vi "Measure-combined.vi"(7 "LaserResponse in":refnum<class "MC-LaserResponse.lvclass">, 8 "error in (no error)":errorcluster, 9 "Device index":i32, 10 "File path":path, 11 "SM1000-control in":T1) -> (0 "error out":errorcluster, 3 "SM1000-control out":T1, 5 "LaserResponse":refnum<class "MC-LaserResponse.lvclass">)   [LabVIEW 2013, in "MaterialCharacterization.lvlib" / "MC-SM1000.lvclass"]
uses:
  MC-SM1000.lvclass
  Object-reference.ctl
  LaserPulseAnalyser/MC-LaserResponse.lvclass
  <vilib>/DAQmx/read.llb/DAQmx Read (Digital 1D U32 1Chan NSamp).vi
  <vilib>/DAQmx/read.llb/DAQmx Read (Analog 2D DBL NChan NSamp).vi
  <vilib>/DAQmx/miscellaneous.llb/DAQmx Fill In Error Info.vi
panel:
  out "Data points":i32
  out "Graph":dbl[][](graph)
  in  "Start job":bool
  out "Job busy":bool
  in  "Stop":bool
  out "Elapsed time":dbl caption="Elapsed time [ms]" format="%.2f"
  out "Initialized":bool
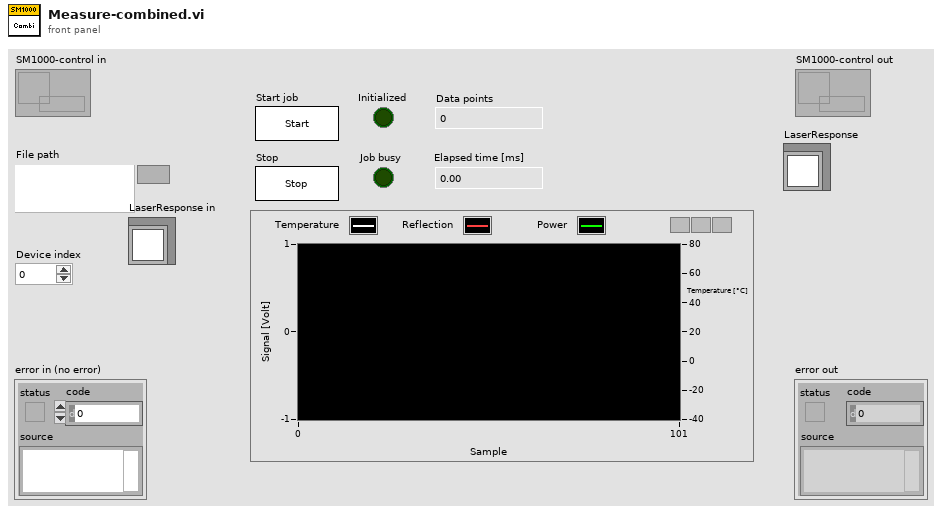
[diagram p1: front panel]
types:
  T1 = typedef "MaterialCharacterization.lvlib/MC-SM1000.lvclass/Object-reference.ctl" = refnum<data-value>
  T2 = enum8{"Enabled", "Disabled", "Disabled and Grayed Out"}
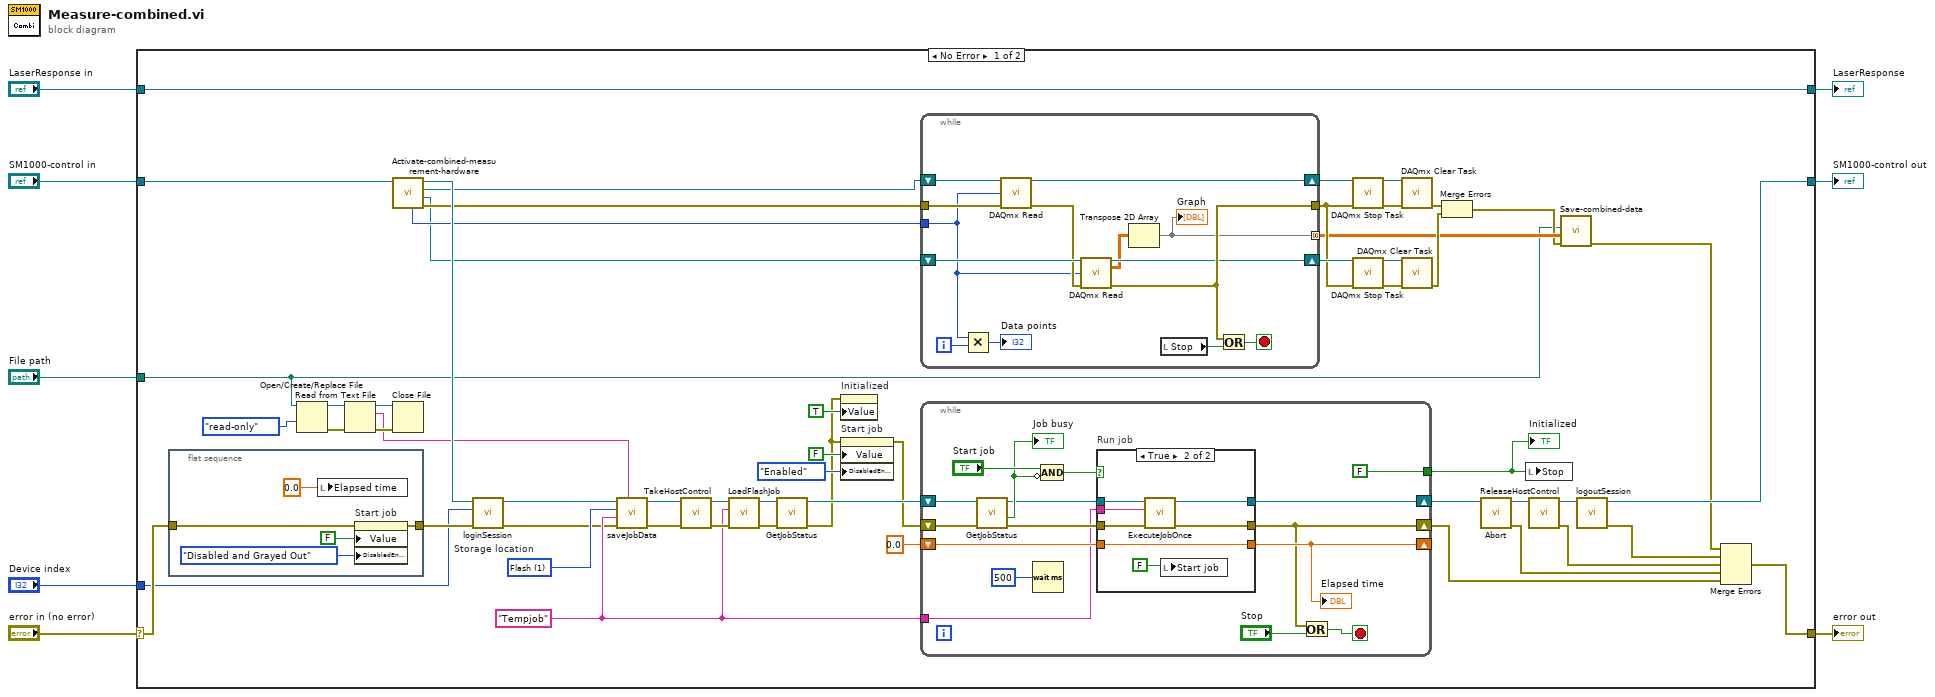
[diagram p0: block diagram]
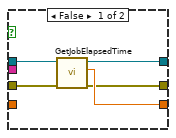
[diagram p2: hidden frame]
diagram:
  n1 = case shown="No Error" "error in (no error)" {
    selector: "error in (no error)" -> [w42 w114]
    tunnel: [w53 w114] -> w7
    tunnel: [w51 w113] -> w5
    tunnel: "SM1000-control in" -> [w38 w113]
    tunnel: "File path" -> [w9 _]
    tunnel: "Device index" -> [w41 _]
    tunnel: "LaserResponse in" -> [w15 w112]
    tunnel: [w15 w112] -> w1
    frame No Error {
      w60 = u16 1 items=["Flash"=1, "USB"=2]  # Storage location
      w57 = "Tempjob"
      n2 = flat-sequence {
        tunnel: [w81] -> w43
        tunnel: w42 -> [w80]
        frame #0 {
          n3 = local write "Elapsed time"(0.0 ("Elapsed time")) -> ()
          n4 = property on="Start job" class="Bool (strict)"(error in=w80, "Value"=FALSE, "DisabledEnum"=T2."Disabled and Grayed Out" ("Disabled")) -> (error out=w81:errorcluster)  [unwired: 1 in, 1 out]
        }
      }
      n5 = Open/Create/Replace File(file path (use dialog)=w9, access (0:read/write)=enum16{"read/write", "read-only", "write-only"}."read-only") -> (refnum out=w16:refnum<file>, error out=w21:errorcluster)  [unwired: 4 in, 1 out]
      n6 = Read from Text File(file (use dialog)=w16, error in=w21) -> (refnum out=w17:refnum<file>, text=w19:string, error out=w22:errorcluster)  [unwired: 2 in, 1 out]
      n7 = call "Activate-combined-measurement-hardware.vi"("SM1000-control in"=w38) -> ("error out"=w14:errorcluster, "Signals"=w13:refnum<k21>, "Control"=w29:refnum<k21>, "SM1000-control out"=w37:T1, "Batch size"=w33:i32)  [unwired: 6 in]
      n8 = Close File(refnum=w17, error in=w22) -> ()  [unwired: 2 out]
      n9 = call "loginSession.vi"("error in (no error)"=w43, "Device index"=w41, "SM1000-control in"=w37) -> ("error out"=w18:errorcluster, "SM1000-control out"=w48:T1)  [unwired: 7 in]
      n10 = call "saveJobData.vi"("Job data xml"=w19, "error in (no error)"=w18, "File name wo extension"=w57, "Storage location"=w60, "SM1000-control in"=w48) -> ("error out"=w35:errorcluster, "SM1000-control out"=w36:T1)  [unwired: 5 in]
      n11 = call "TakeHostControl.vi"("error in (no error)"=w35, "SM1000-control in"=w36) -> ("error out"=w62:errorcluster, "SM1000-control out"=w61:T1)  [unwired: 8 in]
      n12 = call "LoadFlashJob.vi"("error in (no error)"=w62, "Job name wo extension"=w57, "SM1000-control in"=w61) -> ("error out"=w64:errorcluster, "SM1000-control out"=w63:T1)  [unwired: 7 in]
      n13 = call "GetJobStatus.vi"("error in (no error)"=w64, "SM1000-control in"=w63) -> ("error out"=w39:errorcluster, "SM1000-control out"=w59:T1)  [unwired: 7 in, 1 out]
      n14 = property on="Initialized" class="Bool (strict)"(error in=w39, "Value"=TRUE ("Initialized")) -> ()  [unwired: 1 in, 2 out]
      n15 = property on="Start job" class="Bool (strict)"(error in=w39, "Value"=FALSE, "DisabledEnum"=T2."Enabled" ("Disabled")) -> (error out=w47:errorcluster)  [unwired: 1 in, 1 out]
      n16 = while {
        tunnel: w33 -> [w67]
        shift-right: [w76] -> w32
        shift-left: w29 -> [w78]
        shift-right: [w70] -> w27
        shift-left: w13 -> [w73]
        tunnel: w14 -> [w77]
        tunnel: [w71] -> w26
        tunnel: [w65] -> w12 mode=concatenating
        i -> [w69]
        stop <- w75 stop-if-true
        n17 = Multiply(x=w67, y=w69) -> (x*y=→"Data points":i32)
        n18 = call-poly <vilib>:"DAQmx Read.vi"("task/channels in"=w78, "number of samples per channel"=w67, "error in"=w77) -> ("task out"=w76:refnum<k21>, "error out"=w72:errorcluster)  [unwired: 10 in, 1 out]
        n19 = call-poly <vilib>:"DAQmx Read.vi"("task/channels in"=w73, "number of samples per channel"=w67, "error in"=w72) -> ("task out"=w70:refnum<k21>, "data"=w66:dbl[][], "error out"=w71:errorcluster)  [unwired: 10 in]
        n20 = Transpose 2D Array(2D array=w66) -> (transposed array=w65:dbl[][])
        "Graph" <- w65
        n21 = local read "Stop"() -> (w74:bool)
        n22 = Or(x=w71, y=w74) -> (x .or. y?=w75:bool)
      }
      n23 = while {
        shift-right: [w84] -> w34
        shift-left: w47 -> [w98]
        shift-right: [w85] -> w49
        shift-left: w59 -> [w99]
        shift-right: [w89] -> _
        shift-left: 0.0 ("Elapsed time") -> [w90]
        tunnel: w57 -> [w88]
        tunnel: [FALSE] -> w45
        stop <- w93 stop-if-true
        n24 = call "GetJobStatus.vi"("error in (no error)"=w98, "SM1000-control in"=w99) -> ("error out"=w92:errorcluster, "Busy?"=w95:bool, "SM1000-control out"=w91:T1)  [unwired: 7 in]
        "Job busy" <- w95
        n25 = Wait (ms)(milliseconds to wait=u32 500) -> ()  [unwired: 1 out]
        n26 = Compound Arithmetic op=AND("Start job", invert w95) -> (w96:bool)
        n27 = case "Run job" shown="True" w96 {
          tunnel: w92 -> [w102 w108]
          tunnel: [w100 w107] -> w84
          tunnel: [w101 w106] -> w85
          tunnel: w91 -> [w104 w109]
          tunnel: [w103 w111] -> w89
          tunnel: w90 -> [_ w111]
          tunnel: w88 -> [_ w110]
          frame False {
            n28 = call "GetJobElapsedTime.vi"("error in (no error)"=w102, "SM1000-control in"=w104) -> ("error out"=w100:errorcluster, "Elapsed time"=w103:dbl, "SM1000-control out"=w101:T1)  [unwired: 7 in]
          }
          frame True {
            n29 = call "ExecuteJobOnce.vi"("error in (no error)"=w108, "Job name wo extension"=w110, "SM1000-control in"=w109) -> ("error out"=w107:errorcluster, "SM1000-control out"=w106:T1)  [unwired: 7 in]
            n30 = local write "Start job"(FALSE) -> ()
          }
        }
        "Elapsed time" <- w89
        n31 = Or(x=w84, y="Stop") -> (x .or. y?=w93:bool)
      }
      "Initialized" <- w45
      n32 = call <vilib>:"DAQmx Stop Task.vi"("task/channels in"=w32, "error in"=w26) -> ("task out"=w31:refnum<k21>, "error out"=w30:errorcluster)  [unwired: 12 in]
      n33 = call <vilib>:"DAQmx Stop Task.vi"("task/channels in"=w27, "error in"=w26) -> ("task out"=w25:refnum<k21>, "error out"=w28:errorcluster)  [unwired: 12 in]
      n34 = call <vilib>:"DAQmx Clear Task.vi"("task in"=w31, "error in"=w30) -> ("error out"=w24:errorcluster)  [unwired: 13 in]
      n35 = call <vilib>:"DAQmx Clear Task.vi"("task in"=w25, "error in"=w28) -> ("error out"=w23:errorcluster)  [unwired: 13 in]
      n36 = Merge Errors(w24, w23) -> (w11:errorcluster)
      n37 = call "Abort.vi"("SM1000-control in"=w49) -> ("error out"=w54:errorcluster, "SM1000-control out"=w56:T1)  [unwired: 9 in]
      n38 = local write "Stop"(w45) -> ()
      n39 = call "ReleaseHostControl.vi"("SM1000-control in"=w56) -> ("error out"=w55:errorcluster, "SM1000-control out"=w52:T1)  [unwired: 9 in]
      n40 = call "Save-combined-data.vi"("error in (no error)"=w11, "Signal data"=w12, "File path"=w9) -> ("error out"=w10:errorcluster)  [unwired: 8 in]
      n41 = call "logoutSession.vi"("SM1000-control in"=w52) -> ("error out"=w50:errorcluster, "SM1000-control out"=w51:T1)  [unwired: 9 in]
      n42 = Merge Errors(w10, w50, w55, w54, w34) -> (w53:errorcluster)
    }
    frame Error {
    }
  }
  "error out" <- w7
  "SM1000-control out" <- w5
  "LaserResponse" <- w1
